vi "Actor Core.vi"(8 "error in":errorcluster, 11 "LED Matrix in":refnum<class "LED Matrix.lvclass">) -> (0 "error out":errorcluster, 3 "Actor out":refnum<class "Actor.lvclass">)   [LabVIEW 2026, in "LED Matrix.lvlib" / "LED Matrix.lvclass"]
doc: "<p>(<strong>Filename</strong>: <span class=\"dnl\">Actor Framework.lvlib:Actor.lvclass:Actor Core.vi</span>)</p>\n<p>Receives messages to the actor, reacts to them, and initiates any error handling that may shut the actor down.</p>\n<p>Descendant classes may override this VI to append parallel tasks for the actor to complete while it handles messages. Overrides use the <a href=\"nihelplauncher://docs/csh?context=lvcore_glang_udclass\">Call Parent Class Method</a> node.</p>"
uses:
  LED Matrix.lvclass
  <vilib>/ActorFramework/Actor/Actor.lvclass
  LED Matrix.lvclass/LED Matrix.ctl
  Text/Text.lvclass
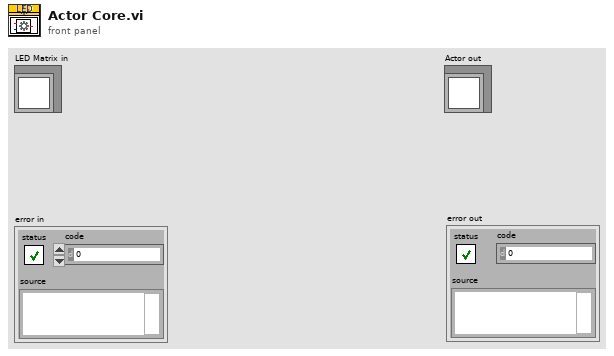
[diagram p1: front panel]
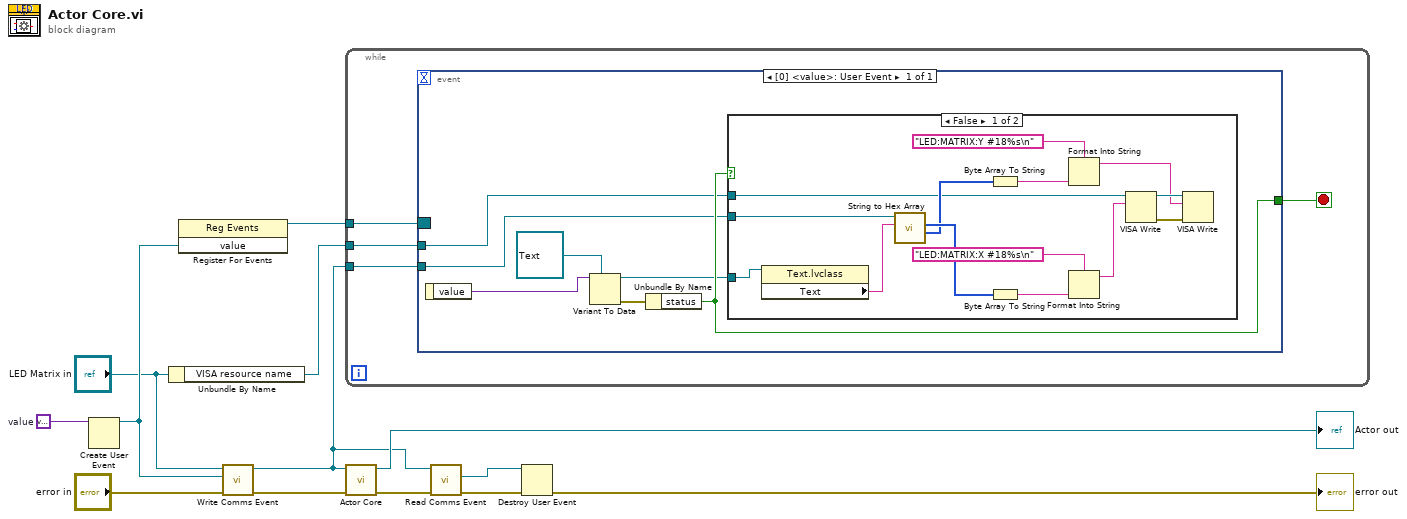
[diagram p0: block diagram]
diagram:
  w6 = variant  # value
  n1 = Create User Event(user event datatype=w6) -> (user event=w10:refnum<user-event>)  [unwired: 1 in, 1 out]
  n2 = Unbundle By Name("LED Matrix in") -> ("VISA resource name"=w7:refnum<visa-resource-name>)
  n3 = register-events(w10) -> (reference out=w9:refnum<event-registration>)  [unwired: 2 in, 1 out]
  n4 = call-dynamic "Write Comms Event.vi"("error in (no error)"="error in", "Comms Event"=w10, "LED Matrix in"="LED Matrix in") -> ("error out"=w11:errorcluster, "LED Matrix out"=w1:refnum<class "LED Matrix.lvclass">)  [unwired: 7 in]
  n5 = while {
    tunnel: w9 -> [w17]
    tunnel: w7 -> [w15]
    tunnel: w1 -> [w14]
    stop <- w16 stop-if-true
    n6 = event shown="[0] <value>: User Event" {
      selector: w17 -> [_]
      dyn-events: _ -> [_]
      timeout: _ -> [_]
      tunnel: [w22] -> w16
      tunnel: w15 -> [w20]
      tunnel: w14 -> [w18]
      event User Event {
        n7 = event-data() -> ("value"=w24:variant)  [unwired: 1 in]
        n8 = Variant To Data(type=refnum<class "Text.lvclass"> refnum ("LED Matrix.lvlib:Text.lvclass"), Variant=w24) -> (data=w21:refnum<class "Text.lvclass">, error out=w23:errorcluster)  [unwired: 1 in]
        n9 = Unbundle By Name(w23) -> ("status"=w22:bool)
        n10 = case shown="False" w22 {
          tunnel: w21 -> [w26 _]
          tunnel: w20 -> [w30 _]
          tunnel: w18 -> [w38 _]
          frame False {
            n11 = property class="Text.lvclass"(reference=w26) -> ("Text"=w25:string)  [unwired: 1 in, 2 out]
            n12 = call "String to Hex Array.vi"("String"=w25, "LED Matrix in"=w38) -> ("Right"=w31:u8[], "Left"=w32:u8[])  [unwired: 6 in, 2 out]
            n13 = Byte Array To String(unsigned byte array=w31) -> (string=w35:string)
            n14 = Byte Array To String(unsigned byte array=w32) -> (string=w33:string)
            n15 = Format Into String(format string="LED:MATRIX:Y #18%s\n" ("concatenated string"), w35) -> (resulting string=w28:string)  [unwired: 2 in, 1 out]
            n16 = Format Into String(format string="LED:MATRIX:X #18%s\n" ("concatenated string"), w33) -> (resulting string=w29:string)  [unwired: 2 in, 1 out]
            n17 = VISA Write(VISA resource name=w30, write buffer=w29) -> (VISA resource name out=w37:refnum<visa-resource-name>, error out=w27:errorcluster)  [unwired: 1 in, 1 out]
            n18 = VISA Write(VISA resource name=w37, write buffer=w28, error in (no error)=w27) -> ()  [unwired: 3 out]
          }
          frame True {
          }
        }
      }
    }
  }
  n19 = call-parent "Actor Core.vi"("error in"=w11, "Actor in"=w1) -> ("error out"=w13:errorcluster, "Actor out"=→"Actor out":refnum<class "Actor.lvclass">)  [unwired: 8 in]
  n20 = call-dynamic "Read Comms Event.vi"("error in (no error)"=w13, "LED Matrix in"=w1) -> ("error out"=w5:errorcluster, "Comms Event"=w2:refnum<user-event>)  [unwired: 7 in, 1 out]
  n21 = Destroy User Event(user event=w2, error in=w5) -> (error out=→"error out":errorcluster)
